vi "FTW-Example-WebSocket-Server-RequestResponse-CustomCallback.vi"() -> ()   [LabVIEW 2015]
panel:
  out "Primary Inbox Address":string="ws://127.0.0.1:65440"
  out "error out":errorcluster
  in  "stop":bool
  out "Request Header Received":string
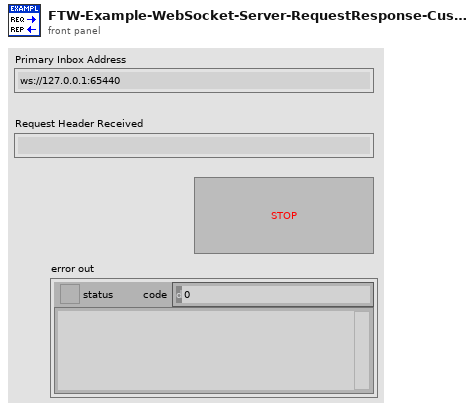
[diagram p1: front panel]
types:
  T1 = typedef "FTW-Type-Actor-Inbox.ctl" = refnum<data-value>
  T2 = typedef "FTW-Type-JSON.ctl" = refnum<data-value>
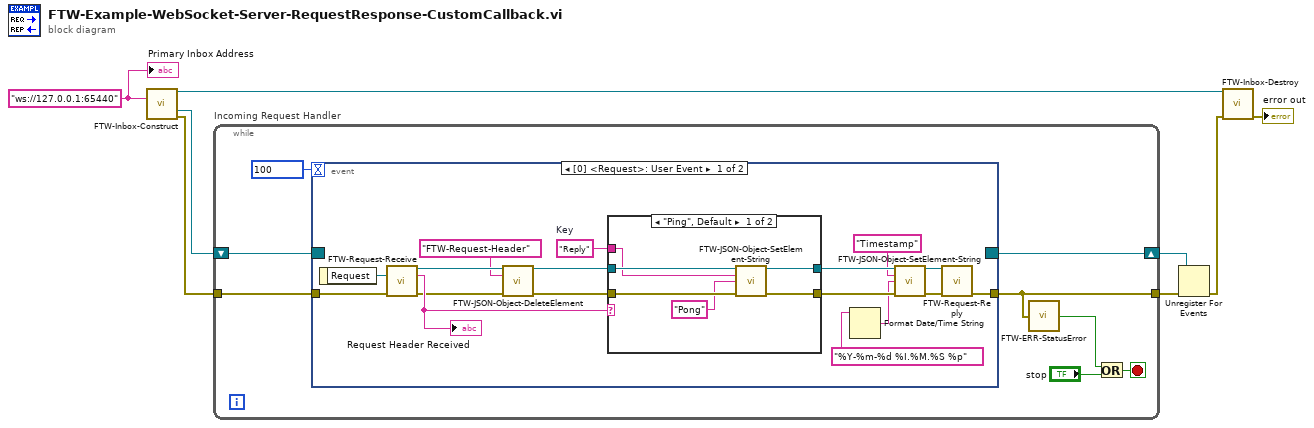
[diagram p0: block diagram]
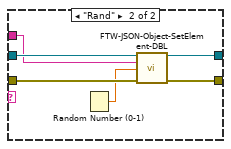
[diagram p2: hidden frame]
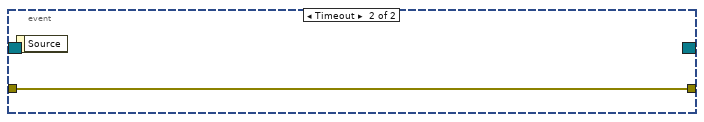
[diagram p3: hidden frame]
diagram:
  w4 = "ws://127.0.0.1:65440" ("Primary Inbox Address")
  n1 = call "FTW-Inbox-Construct.vi"("Primary Inbox Address"=w4) -> ("FTW Actor Inbox"=w1:T1, "Incoming Request"=w6:refnum<event-registration>, "error out"=w5:errorcluster)  [unwired: 9 in, 3 out]
  n2 = while "Incoming Request Handler" {
    shift-right: [w15] -> w7
    shift-left: w6 -> [w16]
    tunnel: w5 -> [w14]
    tunnel: [w13] -> w8
    stop <- w10 stop-if-true
    n3 = event shown="[0] <Request>: User Event" {
      selector: w16 -> [_ _]
      dyn-events: [_ _] -> w15
      timeout: 100 -> [_ _]
      tunnel: w14 -> [w31 w46]
      tunnel: [w33 w46] -> w13
      event User Event {
        w29 = "Reply"  # Key
        n4 = event-data() -> ("Request"=w32:refnum<queue>)  [unwired: 1 in]
        n5 = call "FTW-Request-Receive.vi"("MessagePipe"=w32, "error in"=w31) -> ("Request"=w27:T2, "Request Header"=w30:string, "error out"=w26:errorcluster)  [unwired: 11 in]
        "Request Header Received" <- w30
        n6 = call "FTW-JSON-Object-DeleteElement.vi"("JSON"=w27, "Key"="FTW-Request-Header", "error in"=w26) -> ("JSON out"=w28:T2, "error out"=w25:errorcluster)  [unwired: 10 in, 1 out]
        n7 = case shown="\"Ping\", Default" w30 {
          tunnel: [w36 w42] -> w23
          tunnel: w28 -> [w39 w43]
          tunnel: w25 -> [w38 w44]
          tunnel: [w37 w45] -> w20
          tunnel: w29 -> [w35 w41]
          frame "Ping", Default {
            n8 = call "FTW-JSON-Object-SetElement-String.vi"("JSON"=w39, "Key"=w35, "Value"="Pong", "error in"=w38) -> ("JSON out"=w36:T2, "error out"=w37:errorcluster)  [unwired: 10 in]
          }
          frame "Rand" {
            n9 = Random Number (0-1)() -> (number: 0 to 1=w40:dbl)
            n10 = call "FTW-JSON-Object-SetElement-DBL.vi"("JSON"=w43, "Key"=w41, "Value"=w40, "error in"=w44) -> ("JSON out"=w42:T2, "error out"=w45:errorcluster)  [unwired: 10 in]
          }
        }
        n11 = Format Date/Time String(time format string (%c)="%Y-%m-%d %I.%M.%S %p") -> (date/time string=w18:string)  [unwired: 2 in]
        n12 = call "FTW-JSON-Object-SetElement-String.vi"("JSON"=w23, "Key"="Timestamp", "Value"=w18, "error in"=w20) -> ("JSON out"=w22:T2, "error out"=w21:errorcluster)  [unwired: 10 in]
        n13 = call "FTW-Request-Reply.vi"("Request"=w22, "error in"=w21) -> ("error out"=w33:errorcluster)  [unwired: 13 in]
      }
      event Timeout {
        n14 = event-data() -> ()  [unwired: 1 in, 1 out]
      }
    }
    n15 = call "FTW-ERR-StatusError.vi"("error to check"=w13) -> ("Error?"=w12:bool)
    n16 = Or(x=w12, y="stop") -> (x .or. y?=w10:bool)
  }
  n17 = Unregister For Events(event registration refnum=w7, error in=w8) -> (error out=w3:errorcluster)
  n18 = call "FTW-Inbox-Destroy.vi"("FTW Inbox"=w1, "error in"=w3) -> ("error out"=→"error out":errorcluster)  [unwired: 13 in]
  "Primary Inbox Address" <- w4
